vi "TakePictures.vi"(11 "Image":T1) -> ()   [LabVIEW 2015]
uses:
  <vilib>/vision/Image Controls.llb/IMAQ Image.ctl
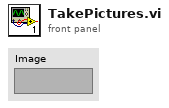
[diagram p1: front panel]
types:
  T1 = typedef "IMAQ Image.ctl" = refnum<image>
  T2 = enum16{"open", "replace", "create", "open or create", "replace or create", "replace or create with confirmation"}
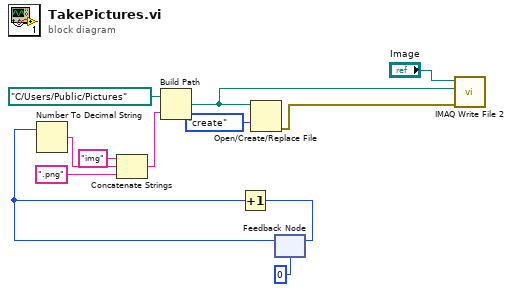
[diagram p0: block diagram]
diagram:
  n1 = feedback #1(0) -> (w5:i32)
  n2 = Number To Decimal String(number=w5) -> (decimal integer string=w9:string)  [unwired: 1 in]
  n3 = Concatenate Strings("img" ("string"), w9, ".png" ("string")) -> (w8:string)
  n4 = Build Path(base path=path "C:/Users/Public/Pictures", name or relative path=w8) -> (appended path=w7:path)
  n5 = Increment(x=w5) -> (x+1=w4:i32)
  n6 = Open/Create/Replace File(file path (use dialog)=w7, operation (0:open)=T2."create") -> (error out=w6:errorcluster)  [unwired: 4 in, 2 out]
  n7 = feedback-in #1(w4) -> ()
  n8 = call-poly "IMAQ Write File 2"("error in (no error)"=w6, "File Path"=w7, "Image"="Image") -> ()  [unwired: 7 in, 2 out]
